vi "Autonomous.vi"   [LabVIEW 2019]
doc: "This VI starts when autonomous period begins, and will automatically be terminated when it ends. You can carry out timed or sensor driven operations directly to I/O or to subsystems without needing to return to the caller."
uses:
  Framework/Robot Global Data.vi
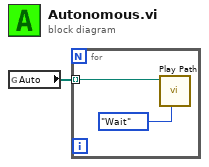
[diagram p0: block diagram]
diagram:
  n1 = global read "Robot Global Data.vi" "Auto"() -> (w1:path[])
  n2 = for {
    tunnel: w1 -> [w3] mode=indexing
    n3 = call "Play Path.vi"("Synchronication"=enum16{"Start", "Wait"}."Wait", "Path"=w3) -> ()  [unwired: 9 in, 1 out]
  }
